vi "Get and Intitialize DIDPID Channel References.vi"(6 "FIFO Name":string, 8 "error in (no error)":errorcluster, 9 "Refs":T4[](array[typedef]) {"Signal Refs" format="%.0x"}, 11 "Item Ref in":T3 format="%.0x") -> (0 "error out":errorcluster, 1 "Write to VS Engine":T1 {"Pairs"."Refs" format="%.0x"}, 2 "Lookup Table":variant, 3 "Item Ref out":T3=18446744073709551615 format="%.0x")   [LabVIEW 2015, in "Diagnostics Addon Engine.lvlib"]
uses:
  Diagnostics Addon Engine.lvlib
  <vilib>/NI Veristand/Custom Device API/Custom Device Item Ref.ctl
  DIDPID Signal VS References.ctl
  Inline Async API/Controls/Write To VS Engine.ctl
  <vilib>/NI Veristand/Custom Device API/Data Reference.ctl
  Datatable Lookup Positions.ctl
  Inline Async API/Inline Async API.lvlib
  <vilib>/NI Veristand/Custom Device API/Custom Device API.lvlib
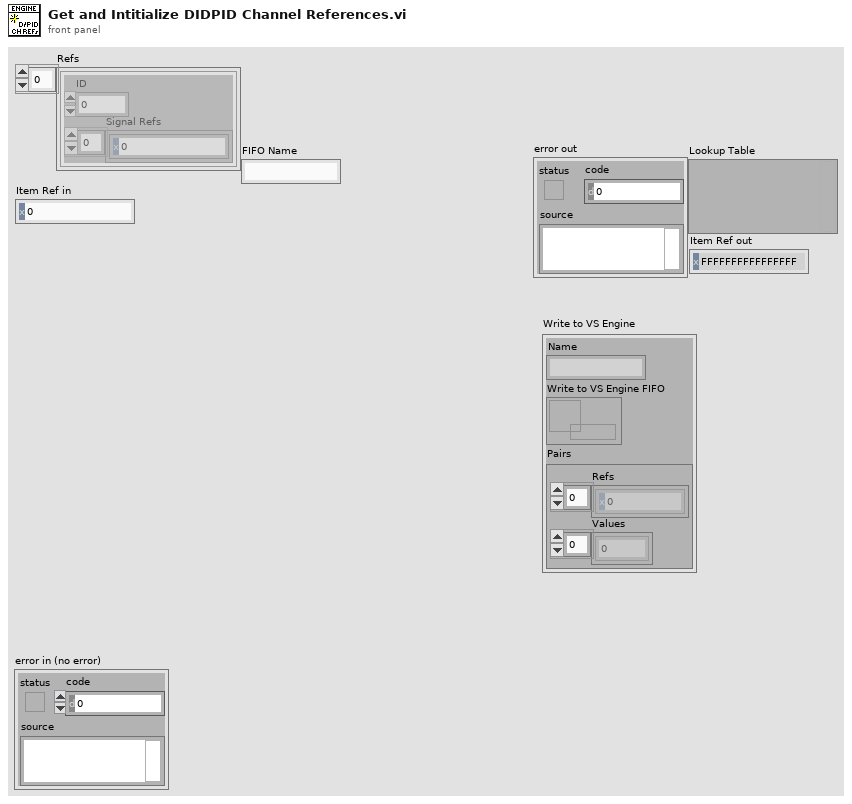
[diagram p1: front panel]
types:
  T1 = typedef "Diagnostics Addon Engine.lvlib/Inline Async API.lvlib/Write To VS Engine.ctl" = cluster{"Name":string, "Write to VS Engine FIFO":refnum<k33>, "Pairs":cluster{"Refs":T2[], "Values":dbl[]}}
  T2 = typedef "Custom Device API.lvlib/Data Reference.ctl" = i32
  T3 = typedef "Custom Device API.lvlib/Custom Device Item Ref.ctl" = u64
  T4 = typedef "Diagnostics Addon Engine.lvlib/DIDPID Signal VS References.ctl" = cluster{"ID":u16, "Signal Refs":T3[]}
  T5 = typedef "Diagnostics Addon Engine.lvlib/Datatable Lookup Positions.ctl" = cluster{"Offset":i32, "Length":i32}
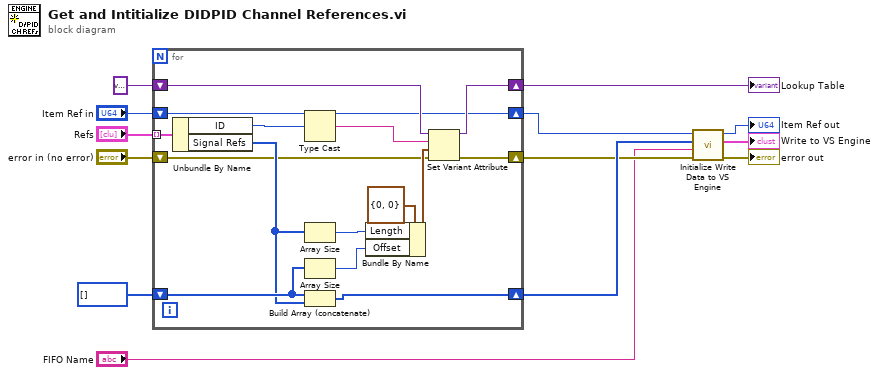
[diagram p0: block diagram]
diagram:
  n1 = for {
    tunnel: "Refs" -> [w18] mode=indexing
    shift-right: [w27] -> w8
    shift-left: T3[] [] ("Signal Refs") -> [w28]
    shift-right: [w19] -> w9
    shift-left: variant -> [w23]
    shift-right: [w21] -> w7
    shift-left: "error in (no error)" -> [w15]
    shift-right: [w14] -> w5
    shift-left: "Item Ref in" -> [w14]
    n2 = Unbundle By Name(w18) -> ("ID"=w17:u16, "Signal Refs"=w16:T3[])
    n3 = Type Cast(x=w17) -> (*(type *) &x=w20:string)  [unwired: 1 in]
    n4 = Array Size(array=w16) -> (size(s)=w26:i32)
    n5 = Array Size(array=w28) -> (size(s)=w22:i32)
    n6 = Build Array (concatenate)(w28, w16) -> (w27:T3[])
    n7 = Bundle By Name(cluster=T5 {"Offset"=0, "Length"=0}, "Length"=w26, "Offset"=w22) -> (w24:T5)
    n8 = Set Variant Attribute(Variant=w23, name=w20, value=w24, error in=w15) -> (Variant out=w19:variant, error out=w21:errorcluster)  [unwired: 1 out]
  }
  "Lookup Table" <- w9
  n9 = call "Initialize Write Data to VS Engine.vi"("error in (no error)"=w7, "FIFO Name"="FIFO Name", "Hardware Output Refs"=w8, "Device Ref"=w5) -> ("error out"=→"error out":errorcluster, "Write to VS Engine"=→"Write to VS Engine":T1, "Device Ref out"=→"Item Ref out":T3)  [unwired: 5 in]
